vi "Cholesky decomposition LABVIEW_v1.1.vi"() -> ()   [LabVIEW 2020]
uses:
  <vilib>/Analysis/Matrix/Datatypes/RealMatrix.ctl
  <vilib>/Analysis/7linalg.llb/Real Cholesky Factorization.vi
  <vilib>/Analysis/7linalg.llb/Real Transpose Matrix.vi
  <vilib>/Analysis/baseanly.llb/Full Cholesky Factorization.vi
  <vilib>/Analysis/baseanly.llb/Full Real Matrix Cholesky Factorization.vi
  <vilib>/Analysis/Matrix/Numeric/Subtract/Subtract - RM,RM.vi
  <vilib>/Analysis/NI_AALPro.lvlib
  <vilib>/Analysis/Matrix/NI_Matrix.lvlib
panel:
  out "sum of error":dbl
  out "appended path":path
  out "error":i32
  out "L LABVIEW-FPGA":sgl[][](array[numeric])
  out "L LABVIEW":T1
  out "A input":dbl[][](array[numeric])
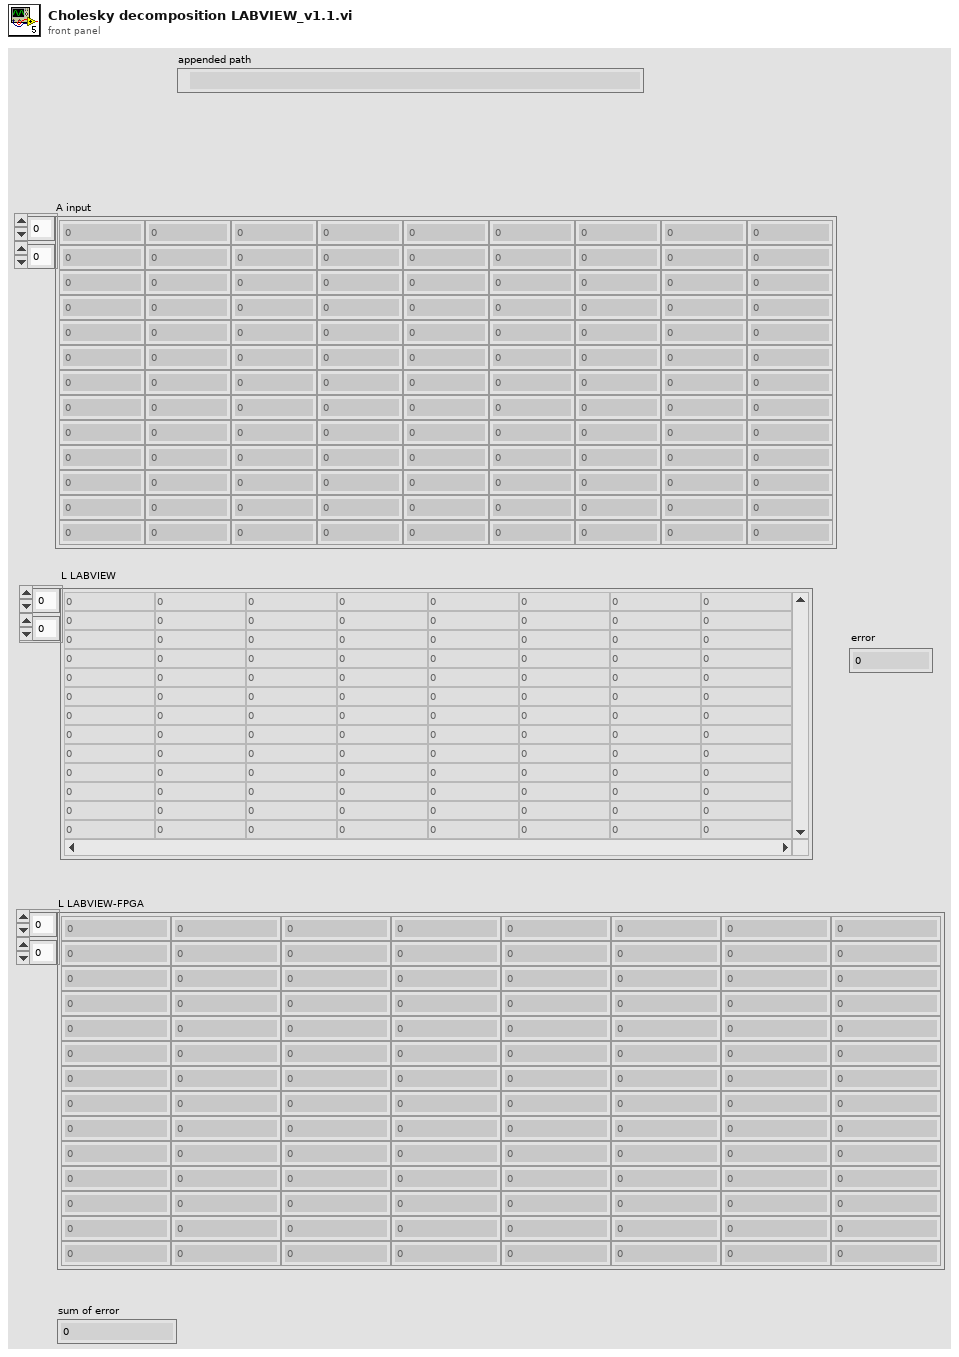
[diagram p1: front panel]
types:
  T1 = typedef "NI_Matrix.lvlib/RealMatrix.ctl" = dbl[][]
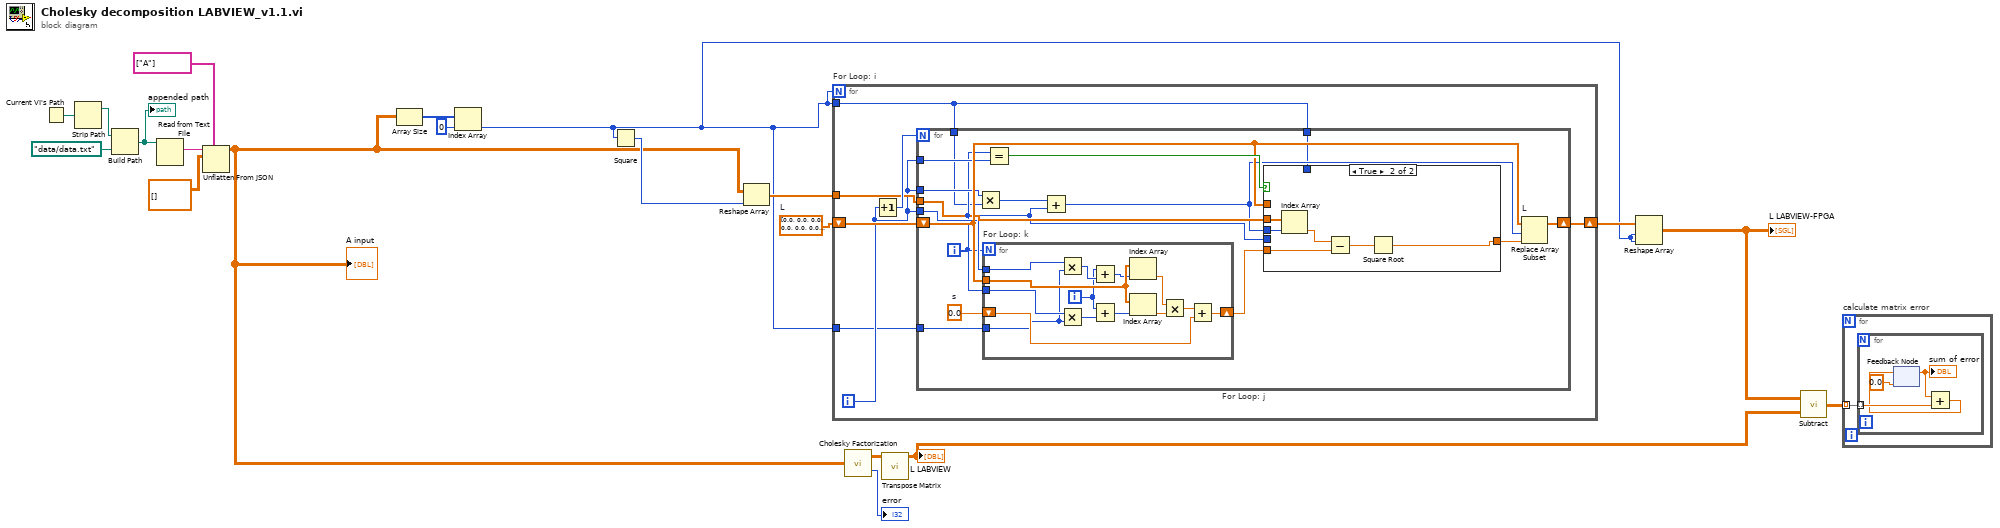
[diagram p0: block diagram]
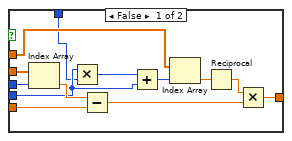
[diagram p2: hidden frame]
diagram:
  w20 = sgl[] [0.0, 0.0, 0.0, 0.0, 0.0, 0.0, 0.0, 0.0, 0.0, 0.0, 0.0, 0.0, 0.0, 0.0, 0.0, 0.0, 0.0, 0.0, 0.0, 0.0, 0.0, 0.0, 0.0, 0.0, 0.0, 0.0, 0.0, 0.0, 0.0, 0.0, 0.0, 0.0, 0.0, 0.0, 0.0, 0.0, 0.0, 0.0, 0.0, 0.0, 0.0, 0.0, 0.0, 0.0, 0.0, 0.0, 0.0, 0.0, 0.0, 0.0, 0.0, 0.0, 0.0, 0.0, 0.0, 0.0, 0.0, 0.0, 0.0, 0.0, 0.0, 0.0, 0.0, 0.0, 0.0, 0.0, 0.0, 0.0, 0.0, 0.0, 0.0, 0.0, 0.0, 0.0, 0.0, 0.0, 0.0, 0.0, 0.0, 0.0, 0.0, 0.0, 0.0, 0.0, 0.0, 0.0, 0.0, 0.0, 0.0, 0.0, 0.0, 0.0, 0.0, 0.0, 0.0, 0.0, 0.0, 0.0, 0.0, 0.0, 0.0, 0.0, 0.0, 0.0, 0.0, 0.0, 0.0, 0.0, 0.0, 0.0, 0.0, 0.0, 0.0, 0.0, 0.0, 0.0, 0.0, 0.0, 0.0, 0.0, 0.0, 0.0, 0.0, 0.0, 0.0, 0.0, 0.0, 0.0, 0.0, 0.0, 0.0, 0.0, 0.0, 0.0, 0.0, 0.0, 0.0, 0.0, 0.0, 0.0, 0.0, 0.0, 0.0, 0.0, 0.0, 0.0, 0.0, 0.0, 0.0, 0.0, 0.0, 0.0, 0.0, 0.0, 0.0, 0.0, 0.0, 0.0, 0.0, 0.0, 0.0, 0.0, 0.0, 0.0, 0.0, 0.0, 0.0, 0.0, 0.0, 0.0, 0.0, 0.0, 0.0, 0.0, 0.0, 0.0, 0.0, 0.0, 0.0, 0.0, 0.0, 0.0, 0.0, 0.0, 0.0, 0.0, 0.0, 0.0, 0.0, 0.0, 0.0, 0.0, 0.0, 0.0, 0.0, 0.0, 0.0, 0.0, 0.0, 0.0, 0.0, 0.0, 0.0, 0.0, 0.0, 0.0, 0.0, 0.0, 0.0, 0.0, 0.0, 0.0, 0.0, 0.0, 0.0, 0.0, 0.0, 0.0, 0.0, 0.0, 0.0, 0.0, 0.0, 0.0, 0.0]  # L
  n1 = Current VI's Path() -> (path=w11:path)
  n2 = Strip Path(path=w11) -> (stripped path=w10:path)  [unwired: 1 out]
  n3 = Build Path(base path=w10, name or relative path=path "data/data.txt") -> (appended path=w12:path)
  "appended path" <- w12
  n4 = Read from Text File(file (use dialog)=w12) -> (text=w16:string)  [unwired: 3 in, 3 out]
  n5 = Unflatten From JSON(path=string[] ["A"], JSON string=w16, type and defaults=dbl[][] []) -> (value=w5:dbl[][])  [unwired: 4 in, 1 out]
  "A input" <- w5
  n6 = Array Size(array=w5) -> (size(s)=w9:i32[])
  n7 = Index Array(array=w9, index=0) -> (element=w6:i32)
  n8 = Square(x=w6) -> (x^2=w7:i32)
  n9 = Reshape Array(w5, w7) -> (w19:dbl[])
  n10 = for "For Loop: i" {
    N: w6 -> [_]
    shift-right: [w25] -> w18
    shift-left: w20 -> [w27]
    tunnel: w19 -> [w24]
    tunnel: w6 -> [w22]
    tunnel: w6 -> [w21]
    i -> [w23]
    n11 = Increment(x=w23) -> (x+1=w26:i32)
    n12 = for "For Loop: j" {
      N: w26 -> [_]
      tunnel: w23 -> [w37]
      shift-right: [w39] -> w25
      shift-left: w27 -> [w38]
      tunnel: w23 -> [w36]
      tunnel: w24 -> [w34]
      tunnel: w23 -> [w32]
      tunnel: w22 -> [w30]
      tunnel: w22 -> [w29]
      tunnel: w21 -> [w28]
      i -> [w31]
      w42 = sgl 0.0  # s
      n13 = Multiply(x=w36, y=w30) -> (x*y=w35:i32)
      n14 = for "For Loop: k" {
        N: w31 -> [_]
        tunnel: w38 -> [w75]
        shift-right: [w71] -> w41
        shift-left: w42 -> [w72]
        tunnel: w32 -> [w70]
        tunnel: w31 -> [w65]
        tunnel: w28 -> [w63]
        i -> [w64]
        n15 = Multiply(x=w70, y=w63) -> (x*y=w69:i32)
        n16 = Multiply(x=w65, y=w63) -> (x*y=w67:i32)
        n17 = Add(x=w64, y=w69) -> (x+y=w68:i32)
        n18 = Add(x=w64, y=w67) -> (x+y=w66:i32)
        n19 = Index Array(array=w75, index=w68) -> (element=w76:sgl)
        n20 = Index Array(array=w75, index=w66) -> (element=w74:sgl)
        n21 = Multiply(x=w76, y=w74) -> (x*y=w73:sgl)
        n22 = Add(x=w73, y=w72) -> (x+y=w71:sgl)
      }
      n23 = Equal?(x=w31, y=w37) -> (x = y?=w43:bool)
      n24 = Add(x=w35, y=w31) -> (x+y=w33:i32)
      n25 = case shown="True" w43 {
        tunnel: w41 -> [w54 w62]
        tunnel: [w53 w60] -> w40
        tunnel: w38 -> [w56 _]
        tunnel: w34 -> [w50 w59]
        tunnel: w33 -> [w49 w58]
        tunnel: w31 -> [w46 _]
        tunnel: w29 -> [w44 _]
        frame False {
          n26 = Index Array(array=w50, index=w49) -> (element=w48:dbl)
          n27 = Multiply(x=w46, y=w44) -> (x*y=w47:i32)
          n28 = Subtract(x=w48, y=w54) -> (x-y=w51:dbl)
          n29 = Add(x=w47, y=w46) -> (x+y=w45:i32)
          n30 = Index Array(array=w56, index=w45) -> (element=w55:sgl)
          n31 = Reciprocal(x=w55) -> (1/x=w52:sgl)
          n32 = Multiply(x=w52, y=w51) -> (x*y=w53:dbl)
        }
        frame True {
          n33 = Index Array(array=w59, index=w58) -> (element=w57:dbl)
          n34 = Subtract(x=w57, y=w62) -> (x-y=w61:dbl)
          n35 = Square Root(x=w61) -> (sqrt(x)=w60:dbl)
        }
      }
      n36 = Replace Array Subset "L"(array=w38, new element=w40, index=w33) -> (w39:sgl[])
    }
  }
  n37 = call-poly <vilib>:"Cholesky Factorization.vi"("A"=w5) -> ("Cholesky"=w4:T1, "error"=→"error":i32)
  n38 = call-poly <vilib>:"Transpose Matrix.vi"("Input Matrix"=w4) -> ("Matrix Transpose"=w1:T1)  [unwired: 9 in, 1 out]
  "L LABVIEW" <- w1
  n39 = Reshape Array(w18, w6, w6) -> (w2:sgl[][])
  "L LABVIEW-FPGA" <- w2
  n40 = call-poly <vilib>:"Subtract.vi"("Real Matrix B"=w1, "Real Matrix A"=w2) -> ("A - B"=w3:T1)
  n41 = for "calculate matrix error" {
    tunnel: w3 -> [w77] mode=indexing
    n42 = for {
      tunnel: w77 -> [w81] mode=indexing
      n43 = feedback #1(0.0) -> (w79:dbl)
      "sum of error" <- w79
      n44 = Add(x=w79, y=w81) -> (x+y=w80:dbl)
      n45 = feedback-in #1(w80) -> ()
    }
  }
